vi "Initialize.vi"(8 "error in (no error)":errorcluster, 9 "GDSII.DataType":refnum<class "GDSII.DataType.lvclass">, 10 "Record Type":string, 11 "Record in":refnum<class "Record.lvclass">) -> (0 "error out":errorcluster, 3 "Record out":refnum<class "Record.lvclass">)   [LabVIEW 2019, in "Record.lvclass"]
uses:
  Record.lvclass
  DataTypes/Base/GDSII.DataType.lvclass
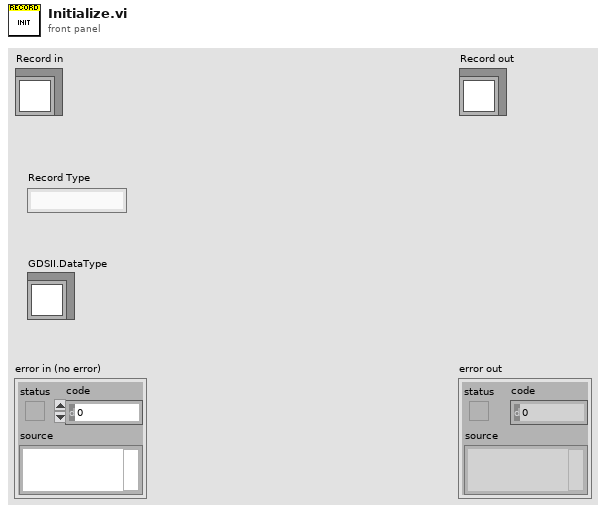
[diagram p1: front panel]
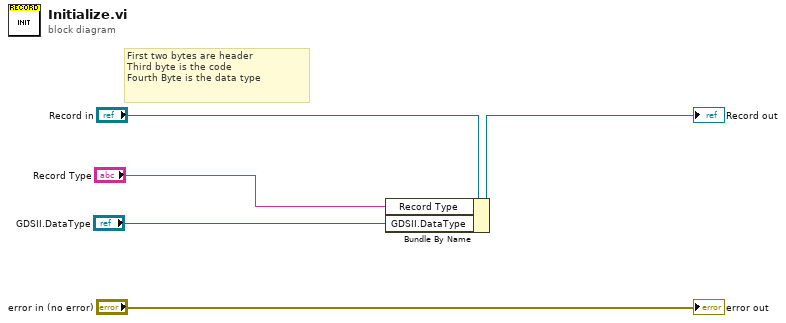
[diagram p0: block diagram]
diagram:
  # "First two bytes are header\nThird byte is the code\nFourth Byte is the data type"
  n1 = Bundle By Name(cluster="Record in", "Record Type"="Record Type", "GDSII.DataType"="GDSII.DataType") -> (→"Record out":refnum<class "Record.lvclass">)
  "error out" <- "error in (no error)"
